vi "array rising edge.vi"(1 "Previous Array":bool[](array[boolean]), 2 "Current Array":bool[](array[boolean])) -> (0 "Update Display":bool)   [LabVIEW 2014]
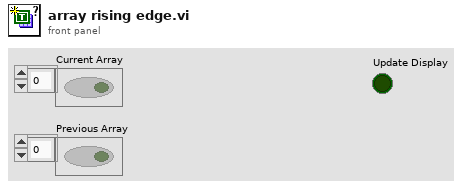
[diagram p1: front panel]
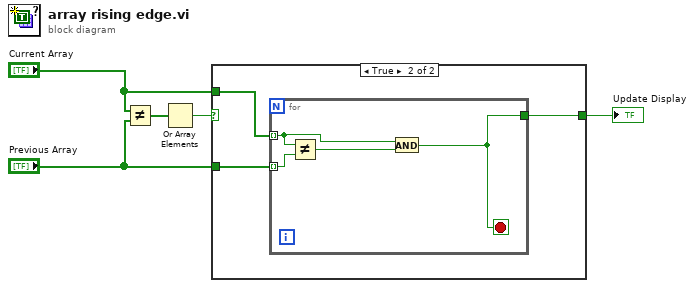
[diagram p0: block diagram]
diagram:
  n1 = Not Equal?(x="Current Array", y="Previous Array") -> (x != y?=w5:bool[])
  n2 = Or Array Elements(Boolean array=w5) -> (logical OR=w4:bool)
  n3 = case shown="True" w4 {
    selector: w4 -> [w6 _]
    tunnel: [w6 w7] -> w3
    tunnel: "Current Array" -> [_ w9]
    tunnel: "Previous Array" -> [_ w8]
    frame False {
    }
    frame True {
      n4 = for {
        tunnel: w9 -> [w11] mode=indexing
        tunnel: w8 -> [w13] mode=indexing
        tunnel: [w10] -> w7
        stop <- w10 stop-if-true
        n5 = Not Equal?(x=w11, y=w13) -> (x != y?=w12:bool)
        n6 = And(x=w11, y=w12) -> (x .and. y?=w10:bool)
      }
    }
  }
  "Update Display" <- w3
